vi "autoSM.vi"(0 "Call Context":T3) -> (1 "Loop 2 SubState":T2=enum."auto", 3 "Loop 2 exit value":i32, 4 "Loop 2 Value 2":dbl, 5 "Loop 3 Value 1":dbl, 7 "Loop 3 Value 2":dbl, 8 "Loop 2 Value 1":dbl, 9 "Loop 3 SubState":T2=enum."auto", 10 "Loop 4 SubState":T2=enum."auto", 11 "Loop 4 exit value":i32, 12 "Loop 0 SubState":T2=enum."auto", 13 "Loop 1 SubState":T2=enum."auto", 14 "Loop 0 exit value":i32, 15 "Loop 1 exit value":i32, 16 "Loop 4 Value 2":dbl, 17 "Loop 3 exit value":i32, 18 "Loop 4 Value 1":dbl, 19 "Pneumatics SubState":T1, 20 "Loop 0 Value 1":dbl, 21 "Loop 5 Exit Value":i32, 22 "Loop 5 Value 2":dbl, 23 "Loop 0 Value 2":dbl, 24 "Loop 1 Value 1":dbl, 26 "Loop 5 Value 1":dbl, 27 "Loop 1 Value 2":dbl)   [LabVIEW 2011]
uses:
  subStates.ctl
  <vilib>/Rock Robotics/WPI/DriverStation/WPI_DriverStationDerivedRobotMode.ctl
  singleUseSubstate.ctl
  fg_typedef.ctl
  vision enable.ctl
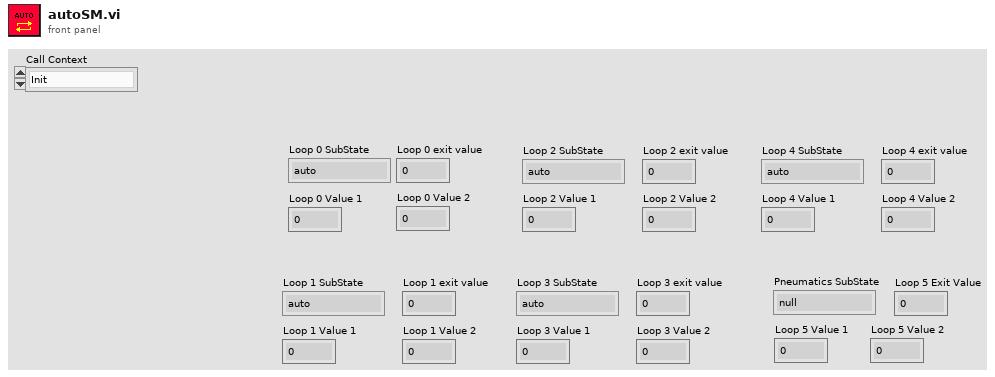
[diagram p1: front panel]
types:
  T1 = typedef "singleUseSubstate.ctl" = enum16{"null", "wait", "shift", "shift high", "shift low", "bridge down", "bridge up", "extender in", "extender out", "extender toggle", "end"}
  T2 = typedef "subStates.ctl" = enum16{"null", "wait", "driver control", "auto", "manual override", "autoDrive", "hold position", "rotate", "end"}
  T3 = typedef "WPI_DriverStationDerivedRobotMode.ctl" = enum16{"Init", "Execute", "Stop"}
  T4 = typedef "vision enable.ctl" = enum16{"Enable", "Disable", "Stop"}
  T5 = typedef "fg_typedef.ctl" = enum16{"Get", "Set"}
  T6 = typedef "WPI_DigitalInputDevRef.ctl" = cluster{"DevStatus":errorcluster, "DIO Channel":T7, "Digital Module":T8}
  T7 = typedef "FPGA_DIOChannel.ctl" = enum8{"DIO 1", "DIO 2", "DIO 3", "DIO 4", "DIO 5", "DIO 6", "DIO 7", "DIO 8", "DIO 9", "DIO 10", "DIO 11", "DIO 12", "DIO 13", "DIO 14", "Invalid"}
  T8 = typedef "FPGA_TypedefDigitalModule.ctl" = enum16{"Digital Module 1", "Digital Module 2"}
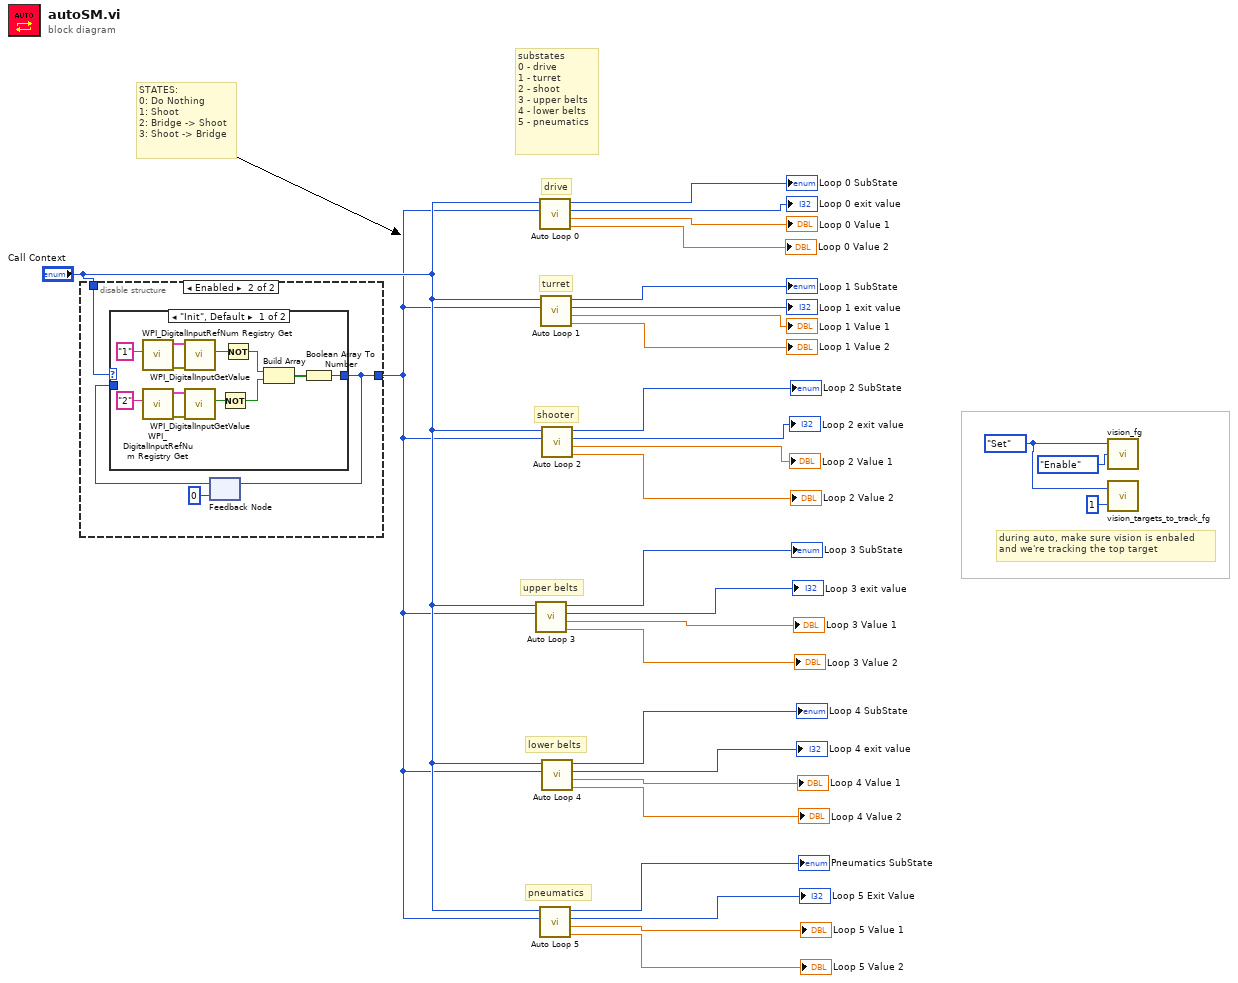
[diagram p0: block diagram]
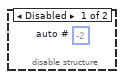
[diagram p2: hidden frame]
diagram:
  w1 = fg_typedef."Set" ("Menu")
  # "during auto, make sure vision is enbaled \nand we're tracking the top target"
  # "pneumatics"
  # "lower belts"
  # "upper belts"
  # "shooter"
  # "turret"
  # "drive"
  # "STATES:\n0: Do Nothing\n1: Shoot\n2: Bridge -> Shoot\n3: Shoot -> Bridge"
  # "substates\n0 - drive\n1 - turret\n2 - shoot\n3 - upper belts\n4 - lower belts\n5 - pneumatics"
  n1 = disable-structure shown="Enabled" {
    disable-tunnel: "Call Context" -> [_ w34]
    disable-tunnel: [_ w31] -> w6
    frame Disabled {
      w30 = -2  # auto #
    }
    frame Enabled {
      n2 = feedback #1(u32 0) -> (w33:u32)
      n3 = case shown="\"Init\", Default" w34 {
        tunnel: [w37 w47] -> w31
        tunnel: w33 -> [_ w47]
        frame "Init", Default {
          n4 = call <vilib>:"WPI_DigitalInputRefNum Registry Get.vi"("refnum name"="1") -> ("error out"=w44:errorcluster, "DigitalInputDevRef"=w43:T6)  [unwired: 9 in]
          n5 = call <vilib>:"WPI_DigitalInputRefNum Registry Get.vi"("refnum name"="2") -> ("error out"=w42:errorcluster, "DigitalInputDevRef"=w41:T6)  [unwired: 9 in]
          n6 = call <vilib>:"WPI_DigitalInputGetValue.vi"("error in (no error)"=w44, "DigitalInputDevRef"=w43) -> ("Value"=w40:bool)  [unwired: 7 in, 2 out]
          n7 = call <vilib>:"WPI_DigitalInputGetValue.vi"("error in (no error)"=w42, "DigitalInputDevRef"=w41) -> ("Value"=w39:bool)  [unwired: 7 in, 2 out]
          n8 = Not(x=w39) -> (.not. x?=w35:bool)
          n9 = Not(x=w40) -> (.not. x?=w36:bool)
          n10 = Build Array(w36, w35) -> (w38:bool[])
          n11 = Boolean Array To Number(Boolean array=w38) -> (number=w37:u32)
        }
        frame "Execute" {
        }
      }
      n12 = feedback-in #1(w31) -> ()
    }
  }
  n13 = call "Auto Loop 3.vi"("auto #"=w6, "Call Context"="Call Context") -> ("Loop 3 Value2"=→"Loop 3 Value 2":dbl, "Loop 3 Value1"=→"Loop 3 Value 1":dbl, "Loop 3 exit value"=→"Loop 3 exit value":i32, "Loop 3 SubState"=→"Loop 3 SubState":T2)  [unwired: 6 in]
  n14 = call "Auto Loop 0.vi"("auto #"=w6, "Call Context"="Call Context") -> ("Loop 0 Value2"=→"Loop 0 Value 2":dbl, "Loop 0 Value1"=→"Loop 0 Value 1":dbl, "Loop 0 exit value"=→"Loop 0 exit value":i32, "Loop 0 SubState"=→"Loop 0 SubState":T2)  [unwired: 6 in]
  n15 = call "Auto Loop 5.vi"("auto #"=w6, "Call Context"="Call Context") -> ("Loop 5 Value2"=→"Loop 5 Value 2":dbl, "Loop 5 Value1"=→"Loop 5 Value 1":dbl, "Loop 5 exit value"=→"Loop 5 Exit Value":i32, "Pneumatics SubState 5"=→"Pneumatics SubState":T1)  [unwired: 6 in]
  n16 = call "Auto Loop 1.vi"("auto #"=w6, "Call Context"="Call Context") -> ("Loop 1 Value2"=→"Loop 1 Value 2":dbl, "Loop 1 Value1"=→"Loop 1 Value 1":dbl, "Loop 1 exit value"=→"Loop 1 exit value":i32, "Loop 1 SubState"=→"Loop 1 SubState":T2)  [unwired: 6 in]
  n17 = call "Auto Loop 2.vi"("auto #"=w6, "Call Context"="Call Context") -> ("Loop 2 Value2"=→"Loop 2 Value 2":dbl, "Loop 2 Value1"=→"Loop 2 Value 1":dbl, "Loop 2 exit value"=→"Loop 2 exit value":i32, "Loop 2 SubState"=→"Loop 2 SubState":T2)  [unwired: 6 in]
  n18 = call "Auto Loop 4.vi"("auto #"=w6, "Call Context"="Call Context") -> ("Loop 4 Value2"=→"Loop 4 Value 2":dbl, "Loop 4 Value1"=→"Loop 4 Value 1":dbl, "Loop 4 exit value"=→"Loop 4 exit value":i32, "Loop 4 SubState"=→"Loop 4 SubState":T2)  [unwired: 6 in]
  n19 = call "vision_fg.vi"("Action"=vision_enable."Enable", "Menu"=w1) -> ()  [unwired: 1 in, 2 out]
  n20 = call "vision_targets_to_track_fg.vi"("Input"=1, "Menu (Get)"=w1) -> ()  [unwired: 1 out]
